vi "Extensions to Browse Pattern.vi"(11 "extensions":string[](array[string])) -> (3 "spreadsheet string":string)   [LabVIEW 2015, in "Engine Simulation Toolkit System Explorer.lvlib"]
uses:
  Engine Simulation Toolkit System Explorer.lvlib
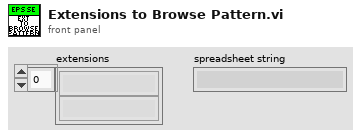
[diagram p1: front panel]
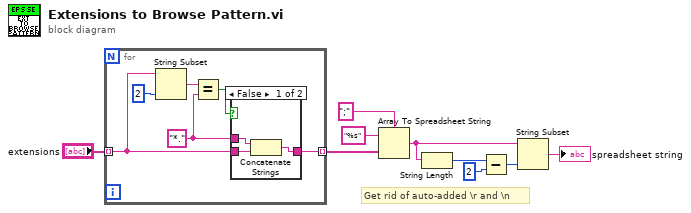
[diagram p0: block diagram]
diagram:
  # "Get rid of auto-added \\r and \\n"
  n1 = for {
    tunnel: "extensions" -> [w14] mode=indexing
    tunnel: [w15] -> w6 mode=indexing
    w11 = "*." ("string")
    n2 = String Subset(string=w14, length (rest)=2 ("length (rest)")) -> (substring=w12:string)  [unwired: 1 in]
    n3 = Equal?(x=w12, y=w11) -> (x = y?=w10:bool)
    n4 = case shown="False" w10 {
      tunnel: [w18 w19] -> w15
      tunnel: w14 -> [w17 w19]
      tunnel: w11 -> [w16 _]
      frame False {
        n5 = Concatenate Strings(w16, w17) -> (w18:string)
      }
      frame True {
      }
    }
  }
  n6 = Array To Spreadsheet String(delimiter (Tab)=";", array=w6, 3:"%s" ("format string")) -> (spreadsheet string=w4:string)
  n7 = String Length(string=w4) -> (length=w3:i32)
  n8 = Subtract(x=w3, y=2) -> (x-y=w1:i32)
  n9 = String Subset(string=w4, length (rest)=w1) -> (substring=→"spreadsheet string":string)  [unwired: 1 in]
